vi "脉冲测量_基于时间_单点.vi"() -> ()   [LabVIEW 2013]
uses:
  <userlib>/ArtDAQ/_SubVI/ArtDAQ_CreateCIPulseChanTime.vi
  <userlib>/ArtDAQ/_SubVI/ArtDAQ_Read Counter Time 1Samp.vi
panel:
  out "低电平时间":dbl
  out "高电平时间":dbl
  in  "Stop":bool
  in  "计数器":string="Dev1/ctr0"
  in  "最小值":dbl format="%0.6f"
  in  "最大值":dbl=1000.0 format="%0.6f"
  out "错误输出":errorcluster
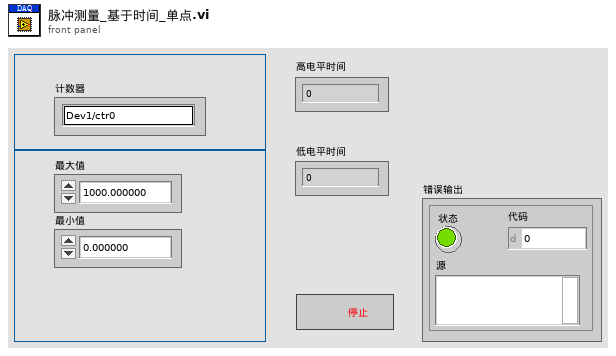
[diagram p1: front panel]
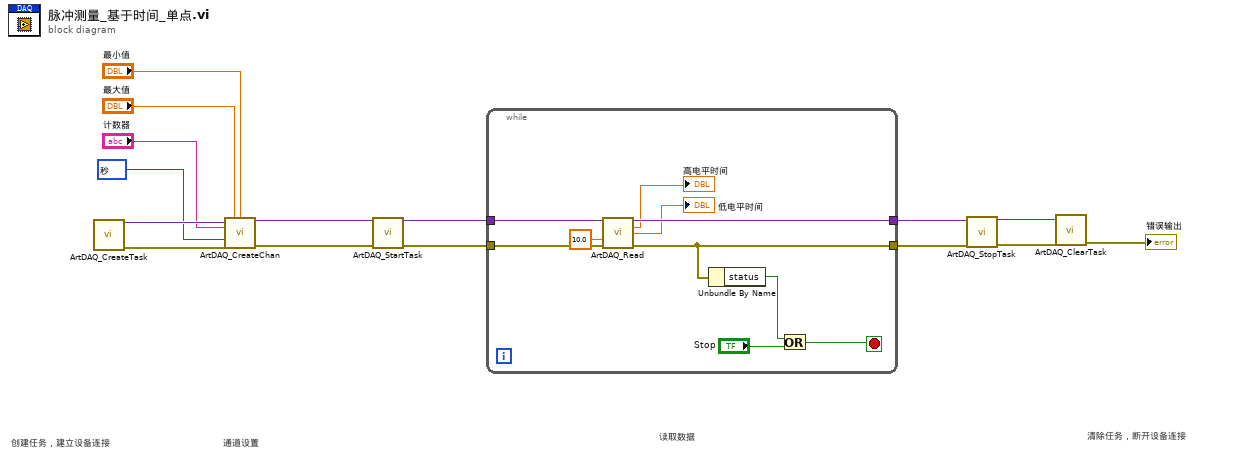
[diagram p0: block diagram]
diagram:
  w5 = 10364 items=["秒"=10364] ("Units")
  # "清除任务，断开设备连接"
  # "读取数据"
  # "通道设置"
  # "创建任务，建立设备连接"
  n1 = call <userlib>:"ArtDAQ_CreateTask.vi"() -> ("任务句柄"=w15:variant, "错误输出"=w14:errorcluster)  [unwired: 14 in]
  n2 = call-poly <userlib>:"ArtDAQ_CreateChan.vi"("任务句柄"=w15, "最大值"="最大值", "最小值"="最小值", "计数器"="计数器", "单位"=w5, "错误输入"=w14) -> ("任务句柄"=w2:variant, "错误输出"=w1:errorcluster)  [unwired: 8 in]
  n3 = call <userlib>:"ArtDAQ_StartTask.vi"("任务句柄"=w2, "错误输入"=w1) -> ("任务句柄"=w4:variant, "错误输出"=w3:errorcluster)  [unwired: 12 in]
  n4 = while {
    tunnel: [w25] -> w12
    tunnel: [w24] -> w10
    tunnel: w4 -> [w20]
    tunnel: w3 -> [w19]
    stop <- w18 stop-if-true
    n5 = call-poly <userlib>:"ArtDAQ_Read.vi"("任务句柄"=w20, "超时s"=10.0 ("Timeout"), "错误输入"=w19) -> ("任务句柄"=w25:variant, "高时间"=→"高电平时间":dbl, "低时间"=→"低电平时间":dbl, "错误输出"=w24:errorcluster)  [unwired: 9 in]
    n6 = Unbundle By Name(w24) -> ("status"=w22:bool)
    n7 = Or(x=w22, y="Stop") -> (x .or. y?=w18:bool)
  }
  n8 = call <userlib>:"ArtDAQ_StopTask.vi"("任务句柄"=w12, "错误输入"=w10) -> ("任务句柄"=w11:variant, "错误输出"=w9:errorcluster)  [unwired: 12 in]
  n9 = call <userlib>:"ArtDAQ_ClearTask.vi"("任务句柄"=w11, "错误输入"=w9) -> ("错误输出"=→"错误输出":errorcluster)  [unwired: 13 in]
